vi "Email Sender.vi"() -> ()   [LabVIEW 2017]
panel:
  in  "Message":string
  in  "Subject":string
  in  "Recipients":string="chyslop@hotmail.co.uk, b8026896@my.shu.ac.uk,"
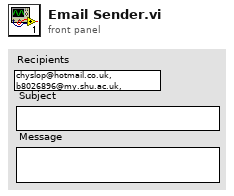
[diagram p1: front panel]
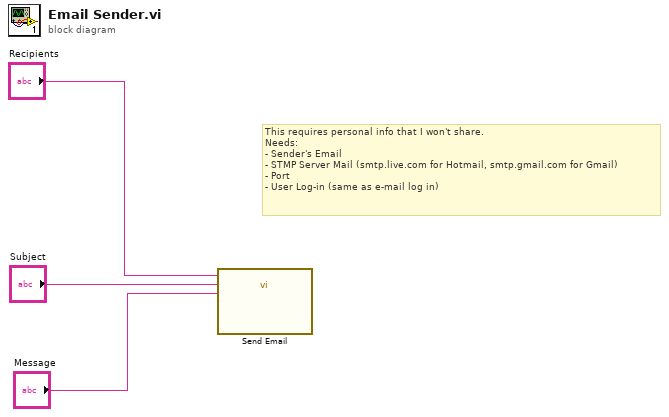
[diagram p0: block diagram]
diagram:
  # "This requires personal info that I won't share.\nNeeds:\n- Sender's Email\n- STMP Server Mail (smtp.live.com for Hotmail, smtp.gmail.com for Gmail)\n- Port\n- User Log-in (same as e-mail log in)"
  n1 = call "Send Email"("Message"="Message", "Subject"="Subject", "Recipients"="Recipients") -> ()  [unwired: 8 in, 1 out]
